vi "Get Monitor Queue.vi"() -> (2 "Caller Enqueuer":refnum<class "Message Enqueuer.lvclass">)   [LabVIEW 2018, in "Monitored Actor.lvlib" / "Actor Monitor.lvclass"]
doc: "GetS the Monitored actor queue ref. If the ref isn't valid, it launches a new instance of the monitor window\n\nCopyright: MGI\nAuthored by: Derek Trepanier"
uses:
  Actor Monitor.lvclass
  <vilib>/ActorFramework/Message Enqueuer/Message Enqueuer.lvclass
  <vilib>/ActorFramework/Message/Message.lvclass
  <vilib>/ActorFramework/Message Enqueuer/Message Enqueuer.lvclass/Message Enqueuer.ctl
  C:/Program Files (x86)/National Instruments/LabVIEW 2018/vi.lib/ActorFramework/Actor/Actor.lvclass
  <vilib>/ActorFramework/Message Queue/Message Queue.lvclass/Message Queue.ctl
  <vilib>/ActorFramework/Message Priority Queue/Priority Enqueue.vi
  <vilib>/ActorFramework/Actor/Actor.lvclass
  <vilib>/ActorFramework/Message Queue/Message Queue.lvclass
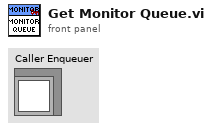
[diagram p1: front panel]
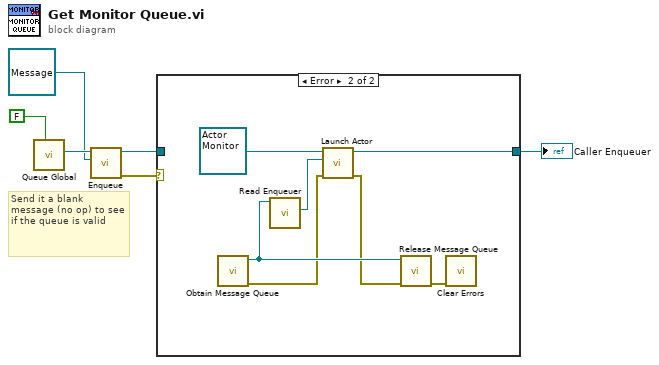
[diagram p0: block diagram]
diagram:
  # "Send it a blank message (no op) to see if the queue is valid"
  n1 = call "Queue Global.vi"("Set?"=FALSE) -> ("Queue out"=w4:refnum<class "Message Enqueuer.lvclass">)  [unwired: 10 in]
  n2 = call <vilib>:"Enqueue.vi"("Message"=refnum<class "Message.lvclass"> refnum, "Message Enqueuer in"=w4) -> ("error out"=w1:errorcluster, "Message Enqueuer out"=w3:refnum<class "Message Enqueuer.lvclass">)  [unwired: 8 in]
  n3 = case shown="Error" w1 {
    tunnel: w3 -> [w7 _]
    tunnel: [w7 w8] -> w5
    frame No Error {
    }
    frame Error {
      n4 = call <vilib>:"Obtain Message Queue.vi"() -> ("error out"=w10:errorcluster, "Message Queue"=w12:refnum<class "Message Queue.lvclass">)  [unwired: 10 in]
      n5 = call <vilib>:"Read Enqueuer.vi"("Message Queue"=w12) -> ("Message Enqueuer"=w13:refnum<class "Message Enqueuer.lvclass">)  [unwired: 10 in]
      n6 = call <vilib>:"Launch Actor.vi"("error in (no error)"=w10, "Actor-to-Caller Enqueuer"=w13, "Actor"=refnum<class "Actor Monitor.lvclass"> refnum ("Monitored Actor.lvlib:Actor Monitor.lvclass")) -> ("error out"=w11:errorcluster, "Caller-To-Actor Enqueuer"=w8:refnum<class "Message Enqueuer.lvclass">)  [unwired: 7 in]
      n7 = call <vilib>:"Release Message Queue.vi"("error in (no error)"=w11, "Message Queue"=w12) -> ("error out"=w9:errorcluster)  [unwired: 8 in, 1 out]
      n8 = call <vilib>:"Clear Errors.vi"("error in (no error)"=w9) -> ()  [unwired: 5 in, 2 out]
    }
  }
  "Caller Enqueuer" <- w5
